vi "triple pll SCTL.vi"(6 "reset":bool, 9 "AI Valid":bool, 10 "AI in":fxp<+/-,16,1>, 11 "param":T1={"base freq (Hz)"=[20123.0, 20123.0, 20123.0], "P gain"=[1234.0, 1234.0, 1234.0], "I gain"=[1.0, 1.0, 1.0], "LP1 coeffs"=[-1025014616, 2098093632, 165702, -1053286467, 2126356551, 167935, -1025014616, 2098093632, 165702, -1053286467, 2126356551, 167935, -1025014616, 2098093632, 165702, -1053286467, 2126356551, 167935], "scope on"=FALSE, "scope channel"=0, "scope signal"=0, "notch coeff"=[-1025014616, 2098093632, 165702, -1053286467, 2126356551, 167935, -1025014616, 2098093632, 165702]}) -> (0 "pulse valid":bool, 1 "3 pulse idx":u32, 2 "phase block valid":bool, 3 "phases out":fxp<+,26,1>[](array[numeric]), 4 "Output Valid":bool, 5 "phase errror mean out":fxp<+,16,1>[](array[numeric]), 7 "freq error mean out":fxp<+/-,16,11>[](array[numeric]))   [LabVIEW 2018, in "SCTL.lvlib"]
uses:
  SCTL.lvlib
  param-sctl-pll.ctl
  <vilib>/rvi/FXPMathLib/FxpSinAndCos/subVIs/nifxpmath_SinAndCos_SimConfig.ctl
  <vilib>/rvi/FXPMathLib/FxpAtan2/subVIs/nifxpmath_Atan2_SimConfig.ctl
  <vilib>/rvi/FXPMathLib/FxpSinAndCos/simVIs/DllFxpSinAndCosTemp_sub.vi
  <vilib>/rvi/FXPMathLib/FxpAtan2/simVIs/DllFxpAtan2Temp_sub.vi
  <vilib>/rvi/FXPMathLib/FxpSinAndCos/XNode/nifxpmath_SinAndCos.xnode
  <vilib>/rvi/FXPMathLib/FxpAtan2/XNode/nifxpmath_Atan2.xnode
  trigger-out.lvlib
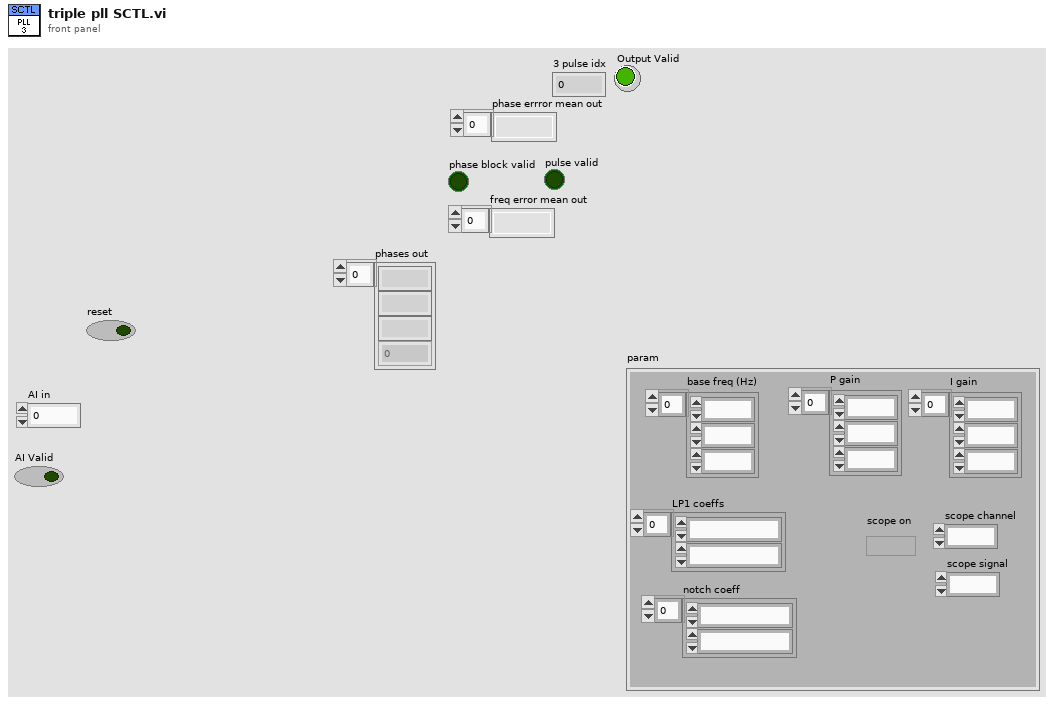
[diagram p1: front panel]
types:
  T1 = typedef "SCTL.lvlib/param-sctl-pll.ctl" = cluster{"base freq (Hz)":fxp<+,17,17>[], "P gain":fxp<+,14,14>[], "I gain":fxp<+,20,6>[], "LP1 coeffs":i32[], "scope on":bool, "scope channel":u8, "scope signal":u8, "notch coeff":i32[]}
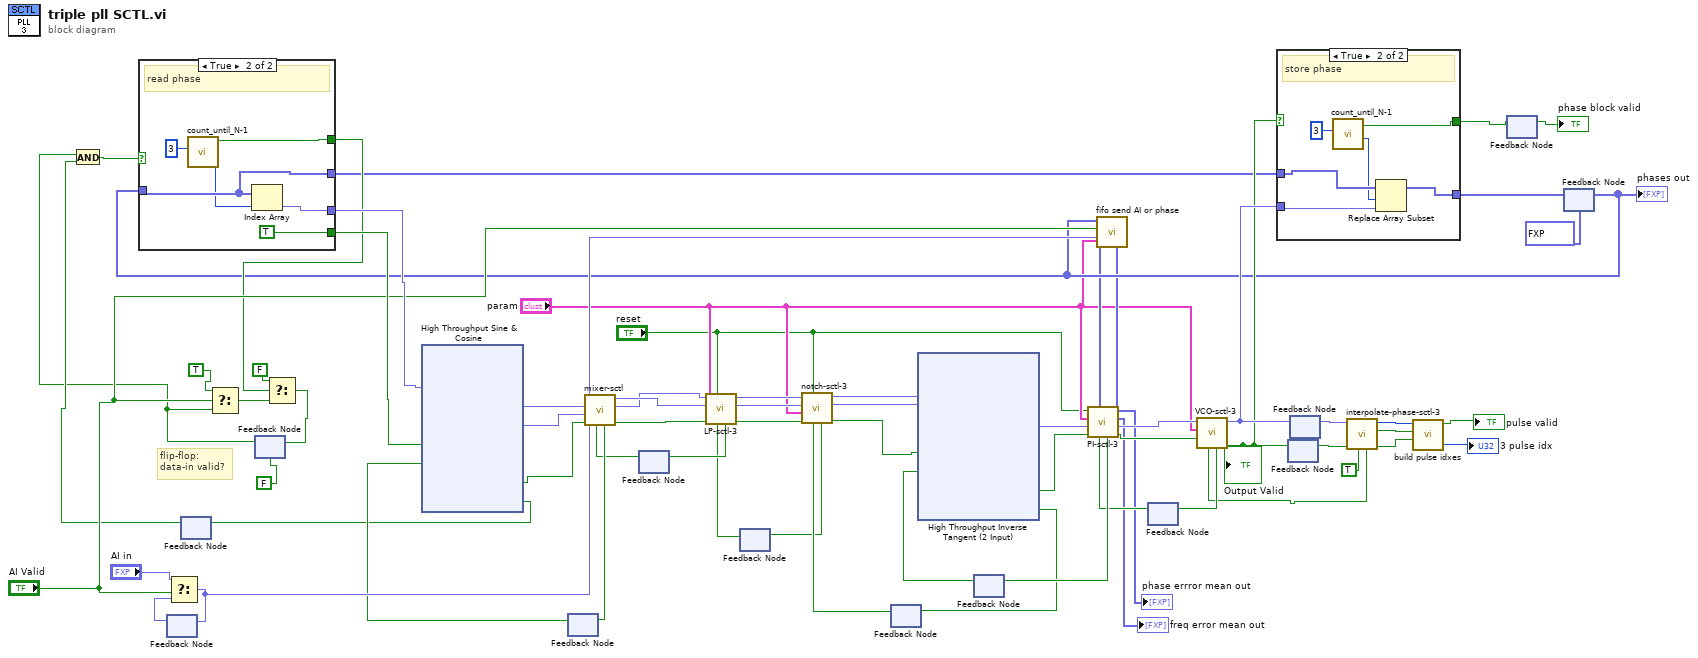
[diagram p0: block diagram]
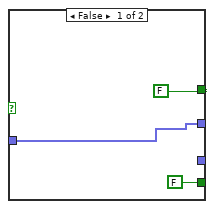
[diagram p2: hidden frame]
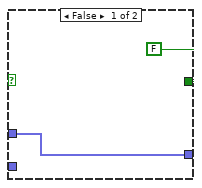
[diagram p3: hidden frame]
diagram:
  # "flip-flop:\ndata-in valid?"
  n1 = feedback #1() -> (w37:fxp<+/-,16,1>)  [unwired: 1 in]
  n2 = Select(t="AI in", s="AI Valid", f=w37) -> (s? t:f=w59:fxp<+/-,16,1>)
  n3 = feedback-in #1(w59) -> ()
  n4 = feedback #2() -> (w30:bool)  [unwired: 1 in]
  n5 = feedback #3(FALSE) -> (w19:bool)
  n6 = And(x=w19, y=w30) -> (x .and. y?=w29:bool)
  n7 = Select(t=TRUE ("input valid"), s="AI Valid", f=w19) -> (s? t:f=w33:bool)
  n8 = feedback #4() -> (w58:bool)  [unwired: 1 in]
  n9 = feedback #5() -> (w61:bool)  [unwired: 1 in]
  n10 = feedback #6() -> (w1:bool)  [unwired: 1 in]
  n11 = feedback #7() -> (w4:bool)  [unwired: 1 in]
  n12 = feedback #8() -> (w67:bool)  [unwired: 1 in]
  n13 = feedback #9() -> (w43:bool)  [unwired: 1 in]
  n14 = feedback #10() -> (w27:bool)  [unwired: 1 in]
  n15 = feedback #11() -> (w28:fxp<+,26,1>)  [unwired: 1 in]
  n16 = call "interpolate-phase-sctl-3.vi"("Ready For Output"=TRUE, "Input Valid"=w27, "phase in"=w28) -> ("Output Valid"=w22:bool, "rising edge!"=w50:bool, "pulse idx out"=w49:u8, "Ready For Input"=w25:bool)  [unwired: 4 in, 1 out]
  n17 = call "build pulse idxes.vi"("Output Valid"=w22, "rising edge!"=w50, "pulse idx in"=w49) -> ("Numeric"=→"3 pulse idx":u32, "Boolean"=→"pulse valid":bool)  [unwired: 7 in]
  n18 = feedback #12() -> (→"phase block valid":bool)  [unwired: 1 in]
  n19 = feedback #13(fxp<+,26,1>[] [0.0, 0.0, 0.0] ("Array")) -> (w16:fxp<+,26,1>[])
  "phases out" <- w16
  n20 = case shown="True" w29 {
    tunnel: [FALSE w72] -> w34
    tunnel: w16 -> [w69 w76]
    tunnel: [w69 w76] -> w20
    tunnel: [_ w75] -> w41
    tunnel: [FALSE ("input valid") TRUE ("input valid")] -> w38
    frame False {
    }
    frame True {
      # "read phase"
      n21 = call "count_until_N-1.vi"("N"=u8 3) -> ("counter"=w71:u8, "turn around !"=w72:bool)  [unwired: 9 in]
      n22 = Index Array(array=w76, index=w71) -> (element=w75:fxp<+,26,1>)
    }
  }
  n23 = Select(t=FALSE ("input valid"), s=w34, f=w33) -> (s? t:f=w31:bool)
  n24 = feedback-in #3(w31) -> ()
  n25 = xnode ("High Throughput Sine & Cosine")("x (pi)"=w41, "input valid"=w38, "ready for output (T)"=w58) -> ("sin(x)"=w66:fxp<+/-,16,2>, "cos(x)"=w65:fxp<+/-,16,2>, "output valid"=w39:bool, "ready for input"=w40:bool)
  n26 = feedback-in #2(w40) -> ()
  n27 = call "mixer-sctl.vi"("Ready For Output"=w61, "Input Valid"=w39, "cos"=w65, "sin"=w66, "AI"=w59) -> ("Output Valid"=w54:bool, "Y"=w52:fxp<+/-,20,2>, "X"=w53:fxp<+/-,20,2>, "Ready For Input"=w64:bool)  [unwired: 3 in]
  n28 = feedback-in #4(w64) -> ()
  n29 = call "LP-sctl-3.vi"("Ready For Output"=w1, "reset"="reset", "Input Valid"=w54, "param"="param", "Y in"=w53, "X in"=w52) -> ("Output Valid"=w3:bool, "Y out"=w10:fxp<+/-,16,1>, "X out"=w11:fxp<+/-,16,1>, "Ready For Input"=w62:bool)  [unwired: 2 in]
  n30 = feedback-in #5(w62) -> ()
  n31 = call "notch-sctl-3.vi"("Ready For Output"=w4, "reset"="reset", "Input Valid"=w3, "param"="param", "Y in"=w10, "X in"=w11) -> ("Output Valid"=w5:bool, "Y out"=w8:fxp<+/-,16,1>, "X out"=w9:fxp<+/-,16,1>, "Ready For Input"=w2:bool)  [unwired: 2 in]
  n32 = feedback-in #6(w2) -> ()
  n33 = xnode ("High Throughput Inverse Tangent (2 Input)")("y"=w9, "x"=w8, "input valid"=w5, "ready for output (T)"=w67) -> ("atan2(y,x) (pi)"=w55:fxp<+/-,16,2>, "output valid"=w24:bool, "ready for input"=w60:bool)
  n34 = feedback-in #7(w60) -> ()
  n35 = call "PI-sctl-3.vi"("Ready For Output"=w43, "Input Valid"=w24, "phase error"=w55, "param"="param", "reset"="reset") -> ("Output Valid"=w45:bool, "freq. error"=w26:fxp<+/-,19,11>, "freq error mean out"=→"freq error mean out":fxp<+/-,16,11>[], "phase errror mean out"=→"phase errror mean out":fxp<+,16,1>[], "Ready For Input"=w63:bool, "freq errors out"=w12:fxp<+/-,16,1>[], "phase errrors out"=w13:fxp<+/-,16,1>[])
  n36 = feedback-in #8(w63) -> ()
  n37 = call "fifo send AI or phase.vi"("freq errors"=w12, "param in"="param", "phase errrors"=w13, "AI in"=w59, "AI Valid in"="AI Valid", "phase"=w16) -> ()  [unwired: 6 in]
  n38 = call "VCO-sctl-3.vi"("Ready For Output"=w25, "Input Valid"=w45, "param"="param", "freq error"=w26) -> ("Output Valid"=w23:bool, "phase"=w51:fxp<+,26,1>, "Ready For Input"=w44:bool)  [unwired: 5 in]
  "Output Valid" <- w23
  n39 = feedback-in #9(w44) -> ()
  n40 = case shown="True" w23 {
    tunnel: w51 -> [_ w84]
    tunnel: [w77 w83] -> w42
    tunnel: [FALSE w79] -> w18
    tunnel: w20 -> [w77 w82]
    frame False {
    }
    frame True {
      # "store phase"
      n41 = call "count_until_N-1.vi"("N"=u8 3) -> ("counter"=w80:u8, "turn around !"=w79:bool)  [unwired: 9 in]
      n42 = Replace Array Subset(array=w82, new element=w84, index=w80) -> (w83:fxp<+,26,1>[])
    }
  }
  n43 = feedback-in #10(w23) -> ()
  n44 = feedback-in #11(w51) -> ()
  n45 = feedback-in #12(w18) -> ()
  n46 = feedback-in #13(w42) -> ()
